vi "Func-엑셀 데이터를 그래프로 출력.vi"() -> ()   [LabVIEW 2015] (continued)
45\t45\t53.083\n45\t45\t53.082\n45\t45\t53.081\n45\t45\t53.079\n45\t45\t53.076\n45\t45\t53.075\n45\t45\t53.074\n45\t45\t53.071\n45\t45\t53.068\n45\t45\t53.065\n45\t45\t53.066\n45\t45\t53.062\n45\t45\t53.059\n45\t45\t53.055\n45\t45\t53.058\n45\t45\t53.057\n45\t45\t53.059\n45\t45\t53.057\n45\t45\t53.059\n45\t45\t53.061\n45\t45\t53.057\n45\t45\t53.056\n45\t45\t53.054\n45\t45\t53.055\n45\t45\t53.052\n45\t45\t53.052\n45\t45\t53.047\n45\t45\t53.045\n45\t45\t53.037\n45\t45\t53.032\n45\t45\t53.03\n45\t45\t53.027\n45\t45\t53.027\n45\t45\t53.027\n45\t45\t53.028\n45\t45\t53.029\n45\t45\t53.03\n45\t45\t53.027\n45\t45\t53.023\n45\t45\t53.021\n45\t45\t53.02\n45\t45\t53.02\n45\t45\t53.018\n45\t45\t53.021\n45\t45\t53.021\n45\t45\t53.023\n45\t45\t53.025\n45\t45\t53.025\n45\t45\t53.023\n45\t45\t53.018\n45\t45\t53.017\n45\t45\t53.012\n45\t45\t53.006\n45\t45\t53.002\n45\t45\t53\n45\t45\t53.003\n45\t45\t53.002\n45\t45\t53\n45\t45\t52.998\n45\t45\t52.996\n45\t45\t52.993\n45\t45\t52.988\n45\t45\t52.984\n45\t45\t52.978\n45\t45\t52.978\n45\t45\t52.975\n45\t45\t52.976\n45\t45\t52.973\n45\t45\t52.975\n45\t45\t52.974\n45\t45\t52.976\n45\t45\t52.976\n45\t45\t52.969\n45\t45\t52.968\n45\t45\t52.966\n45\t45\t52.967\n45\t45\t52.961\n45\t45\t52.96\n45\t45\t52.962\n45\t45\t52.962\n45\t45\t52.957\n45\t45\t52.954\n45\t45\t52.956\n45\t45\t52.955\n45\t45\t52.953\n45\t45\t52.955\n45\t45\t52.953\n45\t45\t52.953\n45\t45\t52.949\n45\t45\t52.947\n45\t45\t52.945\n45\t45\t52.944\n45\t45\t52.946\n45\t45\t52.94\n45\t45\t52.948\n45\t45\t52.947\n45\t45\t52.945\n45\t45\t52.941\n45\t45\t52.939\n45\t45\t52.941\n45\t45\t52.932\n45\t45\t52.929\n45\t45\t52.931\n45\t45\t52.929\n45\t45\t52.928\n45\t45\t52.927\n45\t45\t52.925\n45\t45\t52.927\n45\t45\t52.922\n45\t45\t52.921\n45\t45\t52.921\n45\t45\t52.917\n45\t45\t52.917\n45\t45\t52.915\n45\t45\t52.916\n45\t45\t52.914\n45\t45\t52.909\n45\t45\t52.91\n45\t45\t52.908\n45\t45\t52.907\n45\t45\t52.904\n45\t45\t52.903\n45\t45\t52.901\n45\t45\t52.899\n45\t45\t52.897\n45\t45\t52.896\n45\t45\t52.896\n45\t45\t52.895\n45\t45\t52.895\n45\t45\t52.893\n45\t45\t52.891\n45\t45\t52.891\n45\t45\t52.889\n45\t45\t52.887\n45\t45\t52.887\n45\t45\t52.884\n45\t45\t52.882\n45\t45\t52.879\n45\t45\t52.877\n45\t45\t52.879\n45\t45\t52.875\n45\t45\t52.874\n45\t45\t52.877\n45\t45\t52.877\n45\t45\t52.874\n45\t45\t52.873\n45\t45\t52.875\n45\t45\t52.873\n45\t45\t52.866\n45\t45\t52.862\n45\t45\t52.863\n45\t45\t52.861\n45\t45\t52.856\n45\t45\t52.855\n45\t45\t52.857\n45\t45\t52.856\n45\t45\t52.855\n45\t45\t52.851\n45\t45\t52.85\n45\t45\t52.851\n45\t45\t52.851\n45\t45\t52.854\n45\t45\t52.852\n45\t45\t52.854\n45\t45\t52.851\n45\t45\t52.85\n45\t45\t52.849\n45\t45\t52.844\n45\t45\t52.845\n45\t45\t52.844\n45\t45\t52.843\n45\t45\t52.84\n45\t45\t52.836\n45\t45\t52.835\n45\t45\t52.83\n45\t45\t52.829\n45\t45\t52.828\n45\t45\t52.826\n45\t45\t52.829\n45\t45\t52.826\n45\t45\t52.823\n45\t45\t52.818\n45\t45\t52.817\n45\t45\t52.817\n45\t45\t52.816\n45\t45\t52.814\n45\t45\t52.812\n45\t45\t52.813\n45\t45\t52.812\n45\t45\t52.813\n45\t45\t52.807\n45\t45\t52.808\n45\t45\t52.81\n45\t45\t52.806\n45\t45\t52.809\n45\t45\t52.805\n45\t45\t52.806\n45\t45\t52.803\n45\t45\t52.802\n45\t45\t52.803\n45\t45\t52.8\n45\t45\t52.798\n45\t45\t52.797\n45\t45\t52.799\n45\t45\t52.797\n45\t45\t52.795\n45\t45\t52.792\n45\t45\t52.791\n45\t45\t52.789\n45\t45\t52.786\n45\t45\t52.784\n45\t45\t52.782\n45\t45\t52.788\n45\t45\t52.787\n45\t45\t52.787\n45\t45\t52.786\n45\t45\t52.786\n45\t45\t52.786\n45\t45\t52.778\n45\t45\t52.774\n45\t45\t52.77\n45\t45\t52.766\n45\t45\t52.767\n45\t45\t52.764\n45\t45\t52.764\n45\t45\t52.764\n45\t45\t52.765\n45\t45\t52.766\n45\t45\t52.765\n45\t45\t52.764\n45\t45\t52.759\n45\t45\t52.758\n45\t45\t52.76\n45\t45\t52.756\n45\t45\t52.754\n45\t45\t52.754\n45\t45\t52.755\n45\t45\t52.755\n45\t45\t52.749\n45\t45\t52.748\n45\t45\t52.745\n45\t45\t52.741\n45\t45\t52.743\n45\t45\t52.741\n45\t45\t52.74\n45\t45\t52.739\n45\t45\t52.74\n45\t45\t52.734\n45\t45\t52.738\n45\t45\t52.737\n45\t45\t52.733\n45\t45\t52.734\n45\t45\t52.733\n45\t45\t52.737\n45\t45\t52.734\n45\t45\t52.732\n45\t45\t52.735\n45\t45\t52.732\n45\t45\t52.728\n45\t45\t52.73\n45\t45\t52.723\n45\t45\t52.723\n45\t45\t52.72\n45\t45\t52.72\n45\t45\t52.723\n45\t45\t52.72\n45\t45\t52.721\n45\t45\t52.715\n45\t45\t52.716\n45\t45\t52.713\n45\t45\t52.711\n45\t45\t52.708\n45\t45\t52.707\n45\t45\t52.708\n45\t45\t52.706\n45\t45\t52.706\n45\t45\t52.703\n45\t45\t52.703\n45\t45\t52.705\n45\t45\t52.706\n45\t45\t52.707\n45\t45\t52.702\n45\t45\t52.696\n45\t45\t52.696\n45\t45\t52.692\n45\t45\t52.687\n45\t45\t52.688\n45\t45\t52.693\n45\t45\t52.693\n45\t45\t52.689\n45\t45\t52.69\n45\t45\t52.689\n45\t45\t52.684\n45\t45\t52.68\n45\t45\t52.682\n45\t45\t52.686\n45\t45\t52.684\n45\t45\t52.686\n45\t45\t52.686\n45\t45\t52.684\n45\t45\t52.682\n45\t45\t52.679\n45\t45\t52.677\n45\t45\t52.672\n45\t45\t52.674\n45\t45\t52.672\n45\t45\t52.675\n45\t45\t52.67\n45\t45\t52.672\n45\t45\t52.675\n45\t45\t52.672\n45\t45\t52.671\n45\t45\t52.667\n45\t45\t52.668\n45\t45\t52.665\n45\t45\t52.661\n45\t45\t52.66\n45\t45\t52.661\n45\t45\t52.661\n45\t45\t52.656\n45\t45\t52.654\n45\t45\t52.653\n45\t45\t52.65\n45\t45\t52.648\n45\t45\t52.647\n45\t45\t52.648\n45\t45\t52.652\n45\t45\t52.653\n45\t45\t52.655\n45\t45\t52.654\n45\t45\t52.653\n45\t45\t52.65\n45\t45\t52.647\n45\t45\t52.648\n45\t45\t52.643\n45\t45\t52.641\n45\t45\t52.638\n45\t45\t52.636\n45\t45\t52.635\n45\t45\t52.632\n45\t45\t52.631\n45\t45\t52.631\n45\t45\t52.628\n45\t45\t52.626\n45\t45\t52.627\n45\t45\t52.623\n45\t45\t52.625\n45\t45\t52.623\n45\t45\t52.621\n45\t45\t52.621\n45\t45\t52.618\n45\t45\t52.618\n45\t45\t52.618\n45\t45\t52.618\n45\t45\t52.62\n45\t45\t52.618\n45\t45\t52.618\n45\t45\t52.612\n45\t45\t52.613\n45\t45\t52.61\n45\t45\t52.607\n45\t45\t52.609\n45\t45\t52.609\n45\t45\t52.605\n45\t45\t52.602\n45\t45\t52.602\n45\t45\t52.602\n45\t45\t52.602\n45\t45\t52.604\n45\t45\t52.605\n45\t45\t52.604\n45\t45\t52.603\n45\t45\t52.6\n45\t45\t52.595\n45\t45\t52.591\n45\t45\t52.588\n45\t45\t52.589\n45\t45\t52.589\n45\t45\t52.59\n45\t45\t52.593\n45\t45\t52.589\n45\t45\t52.591\n45\t45\t52.593\n45\t45\t52.589\n45\t45\t52.588\n45\t45\t52.585\n45\t45\t52.588\n45\t45\t52.59\n45\t45\t52.588\n45\t45\t52.59\n45\t45\t52.588\n45\t45\t52.587\n45\t45\t52.59\n45\t45\t52.586\n45\t45\t52.582\n45\t45\t52.577\n45\t45\t52.577\n45\t45\t52.575\n45\t45\t52.569\n45\t45\t52.57\n45\t45\t52.57\n45\t45\t52.571\n45\t45\t52.572\n45\t45\t52.573\n45\t45\t52.572\n45\t45\t52.566\n45\t45\t52.567\n45\t45\t52.562\n45\t45\t52.56\n45\t45\t52.559\n45\t45\t52.559\n45\t45\t52.56\n45\t45\t52.562\n45\t45\t52.565\n45\t45\t52.562\n45\t45\t52.562\n45\t45\t52.559\n45\t45\t52.56\n45\t45\t52.558\n45\t45\t52.555\n45\t45\t52.556\n45\t45\t52.554\n45\t45\t52.555\n45\t45\t52.547\n45\t45\t52.546\n45\t45\t52.546\n45\t45\t52.545\n45\t45\t52.542\n45\t45\t52.539\n45\t45\t52.542\n45\t45\t52.542\n45\t45\t52.54\n45\t45\t52.536\n45\t45\t52.532\n45\t45\t52.533\n45\t45\t52.53\n45\t45\t52.527\n45\t45\t52.528\n45\t45\t52.53\n45\t45\t52.532\n45\t45\t52.53\n45\t45\t52.533\n45\t45\t52.534\n45\t45\t52.531\n45\t45\t52.53\n45\t45\t52.532\n45\t45\t52.53\n45\t45\t52.527\n45\t45\t52.528\n45\t45\t52.522\n45\t45\t52.519\n45\t45\t52.516\n45\t45\t52.516\n45\t45\t52.516\n45\t45\t52.511\n45\t45\t52.516\n45\t45\t52.521\n45\t45\t52.521\n45\t45\t52.521\n45\t45\t52.518\n45\t45\t52.516\n45\t45\t52.514\n45\t45\t52.513\n45\t45\t52.509\n45\t45\t52.507\n45\t45\t52.507\n45\t45\t52.507\n45\t45\t52.505\n45\t45\t52.501\n45\t45\t52.505\n45\t45\t52.503\n45\t45\t52.503\n45\t45\t52.498\n45\t45\t52.496\n45\t45\t52.495\n45\t45\t52.489\n45\t45\t52.492\n45\t45\t52.493\n45\t45\t52.496\n45\t45\t52.496\n45\t45\t52.495\n45\t45\t52.495\n45\t45\t52.491\n45\t45\t52.492\n45\t45\t52.49\n45\t45\t52.491\n45\t45\t52.492\n45\t45\t52.493\n45\t45\t52.495\n45\t45\t52.492\n45\t45\t52.488\n45\t45\t52.489\n45\t45\t52.483\n45\t45\t52.48\n45\t45\t52.479\n45\t45\t52.477\n45\t45\t52.475\n45\t45\t52.473\n45\t45\t52.474\n45\t45\t52.475\n45\t45\t52.476\n45\t45\t52.478\n45\t45\t52.478\n45\t45\t52.475\n45\t45\t52.476\n45\t45\t52.475\n45\t45\t52.473\n45\t45\t52.471\n45\t45\t52.475\n45\t45\t52.477\n45\t45\t52.476\n45\t45\t52.477\n45\t45\t52.479\n45\t45\t52.479\n45\t45\t52.474\n45\t45\t52.474\n45\t45\t52.471\n45\t45\t52.468\n45\t45\t52.462\n45\t45\t52.459\n45\t45\t52.463\n45\t45\t52.46\n45\t45\t52.46\n45\t45\t52.461\n45\t45\t52.461\n45\t45\t52.461\n45\t45\t52.458\n45\t45\t52.455\n45\t45\t52.455\n45\t45\t52.45\n45\t45\t52.449\n45\t45\t52.45\n45\t45\t52.446\n45\t45\t52.446\n45\t45\t52.445\n45\t45\t52.443\n45\t45\t52.442\n45\t45\t52.44\n45\t45\t52.439\n45\t45\t52.436\n45\t45\t52.435\n45\t45\t52.437\n45\t45\t52.436\n45\t45\t52.434\n45\t45\t52.435\n45\t45\t52.438\n45\t45\t52.437\n45\t45\t52.436\n45\t45\t52.437\n45\t45\t52.44\n45\t45\t52.44\n45\t45\t52.435\n45\t45\t52.435\n45\t45\t52.434\n45\t45\t52.43\n45\t45\t52.426\n45\t45\t52.423\n45\t45\t52.424\n45\t45\t52.421\n45\t45\t52.423\n45\t45\t52.423\n45\t45\t52.418\n45\t45\t52.418\n45\t45\t52.419\n45\t45\t52.416\n45\t45\t52.414\n45\t45\t52.414\n45\t45\t52.417\n45\t45\t52.415\n45\t45\t52.411\n45\t45\t52.412\n45\t45\t52.413\n45\t45\t52.412\n45\t45\t52.414\n45\t45\t52.415\n45\t45\t52.418\n45\t45\t52.417\n45\t45\t52.42\n45\t45\t52.418\n45\t45\t52.416\n45\t45\t52.416\n45\t45\t52.412\n45\t45\t52.411\n45\t45\t52.405\n45\t45\t52.403\n45\t45\t52.401\n45\t45\t52.401\n45\t45\t52.403\n45\t45\t52.402\n45\t45\t52.404\n45\t45\t52.404\n45\t45\t52.403\n45\t45\t52.397\n45\t45\t52.393\n45\t45\t52.393\n45\t45\t52.387\n45\t45\t52.388\n45\t45\t52.386\n45\t45\t52.385\n45\t45\t52.384\n45\t45\t52.386\n45\t45\t52.384\n45\t45\t52.382\n45\t45\t52.385\n45\t45\t52.388\n45\t45\t52.389\n45\t45\t52.386\n45\t45\t52.387\n45\t45\t52.386\n45\t45\t52.38\n45\t45\t52.379\n45\t45\t52.373\n45\t45\t52.372\n45\t45\t52.373\n45\t45\t52.37\n45\t45\t52.371\n45\t45\t52.37\n45\t45\t52.375\n45\t45\t52.377\n45\t45\t52.375\n45\t45\t52.379\n45\t45\t52.382\n45\t45\t52.38\n45\t45\t52.373\n45\t45\t52.368\n45\t45\t52.368\n45\t45\t52.368\n45\t45\t52.368\n45\t45\t52.37\n45\t45\t52.374\n45\t45\t52.379\n45\t45\t52.377\n45\t45\t52.371\n45\t45\t52.37\n45\t45\t52.367\n45\t45\t52.362\n45\t45\t52.363\n45\t45\t52.365\n45\t45\t52.37\n45\t45\t52.367\n45\t45\t52.368\n45\t45\t52.365\n45\t45\t52.364\n45\t45\t52.36\n45\t45\t52.357\n45\t45\t52.361\n45\t45\t52.355\n45\t45\t52.361\n45\t45\t52.358\n45\t45\t52.36\n45\t45\t52.359\n45\t45\t52.355\n45\t45\t52.356\n45\t45\t52.348\n45\t45\t52.348\n45\t45\t52.345\n45\t45\t52.341\n45\t45\t52.341\n45\t45\t52.345\n45\t45\t52.347\n45\t45\t52.346\n45\t45\t52.346\n45\t45\t52.35\n45\t45\t52.349\n45\t45\t52.343\n45\t45\t52.341\n45\t45\t52.341\n45\t45\t52.343\n45\t45\t52.339\n45\t45\t52.334\n45\t45\t52.338\n45\t45\t52.338\n45\t45\t52.337\n45\t45\t52.335\n45\t45\t52.335\n45\t45\t52.336\n45\t45\t52.332\n45\t45\t52.333\n45\t45\t52.33\n45\t45\t52.328\n45\t45\t52.327\n45\t45\t52.327\n45\t45\t52.326\n45\t45\t52.323\n45\t45\t52.323\n45\t45\t52.321\n45\t45\t52.319\n45\t45\t52.322\n45\t45\t52.32\n45\t45\t52.323\n45\t45\t52.325\n45\t45\t52.325\n45\t45\t52.327\n45\t45\t52.324\n45\t45\t52.324\n45\t45\t52.32\n45\t45\t52.322\n45\t45\t52.322\n45\t45\t52.321\n45\t45\t52.319\n45\t45\t52.318\n45\t45\t52.32\n45\t45\t52.313\n45\t45\t52.313\n45\t45\t52.313\n45\t45\t52.316\n45\t45\t52.32\n45\t45\t52.319\n45\t45\t52.322\n45\t45\t52.321\n45\t45\t52.315\n45\t45\t52.31\n45\t45\t52.303\n45\t45\t52.299\n45\t45\t52.296\n45\t45\t52.296\n45\t45\t52.299\n45\t45\t52.297\n45\t45\t52.301\n45\t45\t52.305\n45\t45\t52.304\n45\t45\t52.303\n45\t45\t52.301\n45\t45\t52.302\n45\t45\t52.303\n45\t45\t52.299\n45\t45\t52.3\n45\t45\t52.298\n45\t45\t52.298\n45\t45\t52.296\n45\t45\t52.292\n45\t45\t52.29\n45\t45\t52.287\n45\t45\t52.282\n45\t45\t52.284\n45\t45\t52.286\n45\t45\t52.285\n45\t45\t52.282\n45\t45\t52.285\n45\t45\t52.291\n45\t45\t52.287\n45\t45\t52.285\n45\t45\t52.284\n45\t45\t52.287\n45\t45\t52.286\n45\t45\t52.282\n45\t45\t52.282\n45\t45\t52.283\n45\t45\t52.282\n45\t45\t52.28\n45\t45\t52.276\n45\t45\t52.277\n45\t45\t52.278\n45\t45\t52.277\n45\t45\t52.276\n45\t45\t52.277\n45\t45\t52.277\n45\t45\t52.279\n45\t45\t52.273\n45\t45\t52.271\n45\t45\t52.272\n45\t45\t52.271\n45\t45\t52.27\n45\t45\t52.268\n45\t45\t52.273\n45\t45\t52.278\n45\t45\t52.277\n45\t45\t52.274\n45\t45\t52.274\n45\t45\t52.273\n45\t45\t52.27\n45\t45\t52.265\n45\t45\t52.265\n45\t45\t52.265\n45\t45\t52.264\n45\t45\t52.266\n45\t45\t52.264\n45\t45\t52.261\n45\t45\t52.263\n45\t45\t52.261\n45\t45\t52.259\n45\t45\t52.257\n45\t45\t52.258\n45\t45\t52.257\n45\t45\t52.254\n45\t45\t52.253\n45\t45\t52.254\n45\t45\t52.255\n45\t45\t52.254\n45\t45\t52.254\n45\t45\t52.256\n45\t45\t52.258\n45\t45\t52.257\n45\t45\t52.252\n45\t45\t52.254\n45\t45\t52.252\n45\t45\t52.249\n44.917\t44.93\t51.869\n44.833\t44.87\t51.863\n44.75\t44.98\t51.872\n44.667\t44.95\t51.866\n44.583\t44.9\t51.869\n44.5\t44.82\t51.861\n44.417\t44.71\t51.854\n44.333\t44.59\t51.851\n44.25\t44.46\t51.857\n44.167\t44.32\t51.842\n44.083\t44.17\t51.848\n44\t44.02\t51.85\n43.917\t43.88\t51.839\n43.833\t43.72\t51.838\n43.75\t43.57\t51.839\n43.667\t43.41\t51.827\n43.583\t43.26\t51.838\n43.5\t43.12\t51.825\n43.417\t42.99\t51.819\n43.333\t42.87\t51.821\n43.25\t42.75\t51.812\n43.167\t42.64\t51.8\n43.083\t42.55\t51.792\n43\t42.45\t51.785\n42.917\t42.36\t51.772\n42.833\t42.27\t51.77\n42.75\t42.18\t51.767\n42.667\t42.11\t51.749\n42.583\t42.04\t51.743\n42.5\t41.97\t51.723\n42.417\t41.91\t51.714\n42.333\t41.84\t51.7\n42.25\t41.77\t51.689\n42.167\t41.71\t51.668\n42.083\t41.63\t51.662\n42\t41.57\t51.637\n41.917\t41.51\t51.615\n41.833\t41.43\t51.605\n41.75\t41.36\t51.581\n41.667\t41.29\t51.568\n41.583\t41.21\t51.553\n41.5\t41.13\t51.536\n41.417\t41.04\t51.512\n41.333\t40.96\t51.483\n41.25\t40.88\t51.461\n41.167\t40.79\t51.445\n41.083\t40.7\t51.421\n41\t40.61\t51.401\n40.917\t40.52\t51.373\n40.833\t40.45\t51.346\n40.75\t40.36\t51.321\n40.667\t40.27\t51.296\n40.583\t40.18\t51.269\n40.5\t40.1\t51.243\n40.417\t40.01\t51.212\n40.333\t39.91\t51.188\n40.25\t39.83\t51.154\n40.167\t39.75\t51.129\n40.083\t39.65\t51.1\n40\t39.57\t51.07\n39.917\t39.48\t51.039\n39.833\t39.4\t51.001\n39.75\t39.32\t50.979\n39.667\t39.24\t50.937\n39.583\t39.16\t50.902\n39.5\t39.07\t50.88\n39.417\t38.99\t50.843\n39.333\t38.91\t50.797\n39.25\t38.83\t50.77\n39.167\t38.75\t50.737\n39.083\t38.67\t50.698\n39\t38.58\t50.65\n38.917\t38.5\t50.624\n38.833\t38.42\t50.587\n38.75\t38.33\t50.541\n38.667\t38.26\t50.5\n38.583\t38.17\t50.469\n38.5\t38.1\t50.419\n38.417\t38.03\t50.391\n38.333\t37.95\t50.352\n38.25\t37.87\t50.293\n38.167\t37.76\t50.25\n38.083\t37.62\t50.21\n38\t37.45\t50.178\n37.917\t37.3\t50.129\n37.833\t37.15\t50.088\n37.75\t37.01\t50.038\n37.667\t36.86\t50.008\n37.583\t36.74\t49.959\n37.5\t36.65\t49.915\n37.417\t36.58\t49.875\n37.333\t36.54\t49.811\n37.25\t36.51\t49.771\n37.167\t36.5\t49.724\n37.083\t36.52\t49.671\n37\t36.54\t49.626\n36.917\t36.56\t49.575\n36.833\t36.57\t49.527\n36.75\t36.57\t49.48\n36.667\t36.57\t49.434\n36.583\t36.58\t49.381\n36.5\t36.5\t49.334\n36.417\t36.42\t49.267\n36.333\t36.34\t49.23\n36.25\t36.27\t49.174\n36.167\t36.19\t49.123\n36.083\t36.1\t49.075\n36\t36.01\t49.017\n35.917\t35.93\t48.973\n35.833\t35.84\t48.918\n35.75\t35.75\t48.867\n35.667\t35.67\t48.815\n35.583\t35.58\t48.748\n35.5\t35.48\t48.712\n35.417\t35.4\t48.662\n35.333\t35.31\t48.612\n35.25\t35.22\t48.55\n35.167\t35.16\t48.496\n35.083\t34.96\t48.441\n35\t34.84\t48.39\n34.917\t34.75\t48.336\n34.833\t34.65\t48.285\n34.75\t34.57\t48.229\n34.667\t34.47\t48.173\n34.583\t34.4\t48.119\n34.5\t34.31\t48.055\n34.417\t34.23\t48.008\n34.333\t34.15\t47.955\n34.25\t34.07\t47.886\n34.167\t33.99\t47.841\n34.083\t33.91\t47.777\n34\t33.84\t47.718\n33.917\t33.77\t47.666\n33.833\t33.69\t47.609\n33.75\t33.61\t47.56\n33.667\t33.53\t47.489\n33.583\t33.46\t47.436\n33.5\t33.39\t47.381\n33.417\t33.3\t47.321\n33.333\t33.22\t47.267\n33.25\t33.14\t47.197\n33.167\t33.05\t47.134\n33.083\t32.96\t47.089\n33\t32.88\t47.016\n32.917\t32.8\t46.967\n32.833\t32.72\t46.9\n32.75\t32.63\t46.837\n32.667\t32.54\t46.776\n32.583\t32.46\t46.717\n32.5\t32.37\t46.645\n32.417\t32.3\t46.596\n32.333\t32.21\t46.538\n32.25\t32.12\t46.468\n32.167\t32.04\t46.414\n32.083\t31.95\t46.34\n32\t31.87\t46.284\n31.917\t31.78\t46.213\n31.833\t31.7\t46.163\n31.75\t31.61\t46.088\n31.667\t31.53\t46.024\n31.583\t31.45\t45.969\n31.5\t31.37\t45.905\n31.417\t31.29\t45.841\n31.333\t31.2\t45.777\n31.25\t31.12\t45.715\n31.167\t31.03\t45.65\n31.083\t30.94\t45.586\n31\t30.85\t45.519\n30.917\t30.78\t45.45\n30.833\t30.7\t45.376\n30.75\t30.61\t45.318\n30.667\t30.53\t45.26\n30.583\t30.45\t45.198\n30.5\t30.37\t45.12\n30.417\t30.3\t45.056\n30.333\t30.22\t44.991\n30.25\t30.13\t44.909\n30.167\t30.06\t44.856\n30.083\t29.97\t44.782\n30\t29.89\t44.722\n29.917\t29.81\t44.654\n29.833\t29.74\t44.59\n29.75\t29.66\t44.518\n29.667\t29.58\t44.449\n29.583\t29.5\t44.381\n29.5\t29.42\t44.316\n29.417\t29.34\t44.263\n29.333\t29.27\t44.175\n29.25\t29.2\t44.114\n29.167\t29.11\t44.031\n29.083\t29.03\t43.975\n29\t28.94\t43.901\n28.917\t28.86\t43.838\n28.833\t28.78\t43.768\n28.75\t28.7\t43.701\n28.667\t28.62\t43.63\n28.583\t28.54\t43.563\n28.5\t28.46\t43.489\n28.417\t28.38\t43.422\n28.333\t28.3\t43.346\n28.25\t28.23\t43.285\n28.167\t28.14\t43.207\n28.083\t28.05\t43.14\n28\t27.98\t43.071\n27.917\t27.9\t43.002\n27.833\t27.82\t42.921\n27.75\t27.75\t42.858\n27.667\t27.66\t42.789\n27.583\t27.58\t42.716\n27.5\t27.49\t42.649\n27.417\t27.4\t42.571\n27.333\t27.32\t42.51\n27.25\t27.23\t42.436\n27.167\t27.15\t42.36\n27.083\t27.07\t42.289\n27\t26.99\t42.227\n26.917\t26.9\t42.153\n26.833\t26.81\t42.081\n26.75\t26.73\t41.999\n26.667\t26.65\t41.937\n26.583\t26.57\t41.866\n26.5\t26.49\t41.784\n26.417\t26.4\t41.715\n26.333\t26.32\t41.636\n26.25\t26.23\t41.572\n26.167\t26.16\t41.494\n26.083\t26.08\t41.427\n26\t26\t41.356\n25.917\t25.92\t41.278\n25.833\t25.85\t41.208\n25.75\t25.76\t41.131\n25.667\t25.67\t41.064\n25.583\t25.59\t40.984\n25.5\t25.51\t40.914\n25.417\t25.43\t40.841\n25.333\t25.34\t40.767\n25.25\t25.25\t40.697\n25.167\t25.17\t40.62\n25.083\t25.09\t40.551\n25\t25\t40.479\n25\t24.93\t40.406\n25\t24.93\t40.403\n25\t24.93\t40.4\n25\t24.92\t40.388\n25\t24.91\t40.38\n25\t24.9\t40.375\n25\t24.89\t40.369\n25\t24.89\t40.364\n25\t24.88\t40.357\n25\t24.87\t40.345\n25\t24.86\t40.339\n25\t24.85\t40.331\n25\t24.84\t40.322\n25\t24.83\t40.312\n25\t24.82\t40.304\n25\t24.82\t40.299\n25\t24.81\t40.292\n25\t24.8\t40.283\n25\t24.8\t40.278\n25\t24.79\t40.275\n25\t24.78\t40.27\n25\t24.77\t40.26\n25\t24.76\t40.252\n25\t24.75\t40.248\n25\t24.75\t40.24\n25\t24.74\t40.234\n25\t24.73\t40.227\n25\t24.72\t40.221\n25\t24.71\t40.215\n25\t24.71\t40.209\n25\t24.71\t40.198\n25\t24.7\t40.191\n25\t24.69\t40.185\n25\t24.69\t40.171\n25\t24.68\t40.165\n25\t24.67\t40.155\n25\t24.66\t40.143\n25\t24.65\t40.135\n25\t24.65\t40.13\n25\t24.64\t40.123\n25\t24.63\t40.113\n25\t24.62\t40.109\n25\t24.62\t40.104\n25\t24.62\t40.098\n25\t24.61\t40.089\n25\t24.61\t40.086\n25\t24.6\t40.082\n25\t24.59\t40.077\n25\t24.59\t40.07\n25\t24.58\t40.064\n25\t24.58\t40.052\n25\t24.57\t40.045\n25\t24.57\t40.038\n25\t24.56\t40.024\n25\t24.56\t40.021\n25\t24.55\t40.014\n25\t24.55\t40.006\n25\t24.54\t39.997\n25\t24.54\t39.988\n25\t24.54\t39.981\n25\t24.54\t39.968\n25\t24.53\t39.96\n25\t24.53\t39.952\n25\t24.53\t39.946\n25\t24.53\t39.939\n25\t24.53\t39.929\n25\t24.52\t39.923\n25\t24.52\t39.918\n25\t24.52\t39.911\n25\t24.52\t39.901\n25\t24.52\t39.896\n25\t24.52\t39.887\n25\t24.51\t39.885\n25\t24.51\t39.877\n25\t24.51\t39.868\n25\t24.51\t39.863\n25\t24.51\t39.858\n25\t24.51\t39.845\n25\t24.51\t39.837\n25\t24.51\t39.828\n25\t24.5\t39.823\n25\t24.5\t39.817\n25\t24.5\t39.807\n25\t24.51\t39.806\n25\t24.51\t39.796\n25\t24.5\t39.791\n25\t24.51\t39.781\n25\t24.5\t39.773\n25\t24.5\t39.762\n25\t24.5\t39.753\n25\t24.5\t39.75\n25\t24.5\t39.739\n25\t24.5\t39.734\n25\t24.49\t39.725\n25\t24.5\t39.721\n25\t24.5\t39.714\n25\t24.5\t39.704\n25\t24.49\t39.694\n25\t24.49\t39.685\n25\t24.49\t39.685\n25\t24.5\t39.673\n25\t24.5\t39.668\n25\t24.5\t39.66\n25\t24.5\t39.656\n25\t24.5\t39.648\n25\t24.5\t39.636\n25\t24.5\t39.629\n25\t24.51\t39.623\n25\t24.51\t39.616\n25\t24.51\t
